vi "ComputeFontScaleFromRequiredHeight(TextDrawSettings).vi"(6 "Thickness (Default: 1)":i32=1, 7 "Text Drawing Settings in (Default: Simplex)":T1={"OpenCV Font Face"=enum."FONT_HERSHEY_SIMPLEX", "Font Scale"=1.0}, 8 "error in (no error)":errorcluster, 11 "Required Text Height":u16) -> (0 "error out":errorcluster, 5 "Text Drawing Settings out":T1)   [LabVIEW 2020, in "g_ar_toolkit.image.lvlib"]
uses:
  g_ar_toolkit.image.lvlib
  Text Drawing Settings.ctl
  Font Face.ctl
  <vilib>/Utility/error.llb/Error Cluster From Error Code.vi
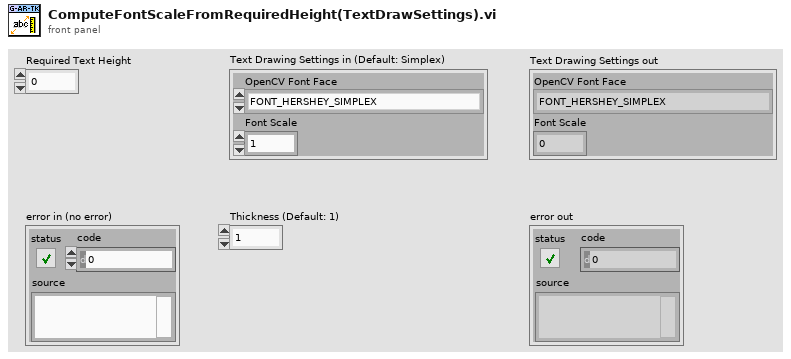
[diagram p1: front panel]
types:
  T1 = typedef "g_ar_toolkit.image.lvlib/Text Drawing Settings.ctl" = cluster{"OpenCV Font Face":T2, "Font Scale":dbl}
  T2 = typedef "g_ar_toolkit.image.lvlib/Font Face.ctl" = enum16{"FONT_HERSHEY_SIMPLEX", "FONT_HERSHEY_PLAIN", "FONT_HERSHEY_DUPLEX", "FONT_HERSHEY_COMPLEX", "FONT_HERSHEY_TRIPLEX", "FONT_HERSHEY_COMPLEX_SMALL", "FONT_HERSHEY_SCRIPT_SIMPLEX", "FONT_HERSHEY_SCRIPT_COMPLEX", "FONT_ITALIC"}
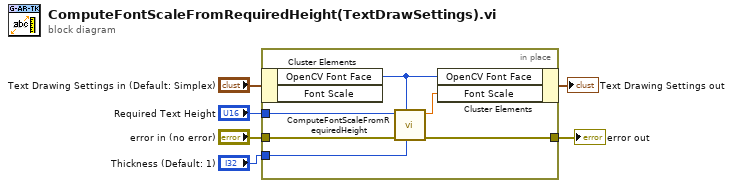
[diagram p0: block diagram]
diagram:
  n1 = in-place {
    in-place-border: "Required Text Height" -> [w12]
    in-place-border: "Thickness (Default: 1)" -> [w11]
    in-place-border: "error in (no error)" -> [w8]
    in-place-border: [w7] -> w2
    n2 = in-place-cluster #1("Text Drawing Settings in (Default: Simplex)") -> ("OpenCV Font Face"=w9:T2)  [unwired: 1 out]
    n3 = call "ComputeFontScaleFromRequiredHeight.vi"("Thickness (Default: 1)"=w11, "OpenCV Font Face"=w9, "error in (no error)"=w8, "Required Text Height"=w12) -> ("error out"=w7:errorcluster, "Font Scale"=w10:dbl)  [unwired: 6 in]
    n4 = in-place-cluster #1("OpenCV Font Face"=w9, "Font Scale"=w10) -> (→"Text Drawing Settings out":T1)
  }
  "error out" <- w2
